vi "Overlay Geometric Pattern Matching Results.vi"(6 "Color":u32(colorbox)=16711680, 7 "Group":string, 8 "error in":errorcluster, 10 "Matches":T2[](array[typedef]) {"Correlation Score" format="%.2f"; "Target Template Curve Score" format="%.2f"; "Template Target Curve Score" format="%.2f"; "Bounding Box"."y" format="%.2f"; "Bounding Box"."x" format="%.2f"; "Position"."y" format="%.2f"; "Position"."x" format="%.2f"; "Score" format="%.2f"; "Scale" format="%.2f"; "Angle" format="%.2f"; "Occlusion %" format="%.2f"}, 11 "Image":T1) -> (0 "error out":errorcluster, 3 "Image Out":T1)   [LabVIEW 2014]
uses:
  <vilib>/vision/Pattern Matching.llb/IMAQ GM Match Report.ctl
  <vilib>/vision/Image Controls.llb/IMAQ Image.ctl
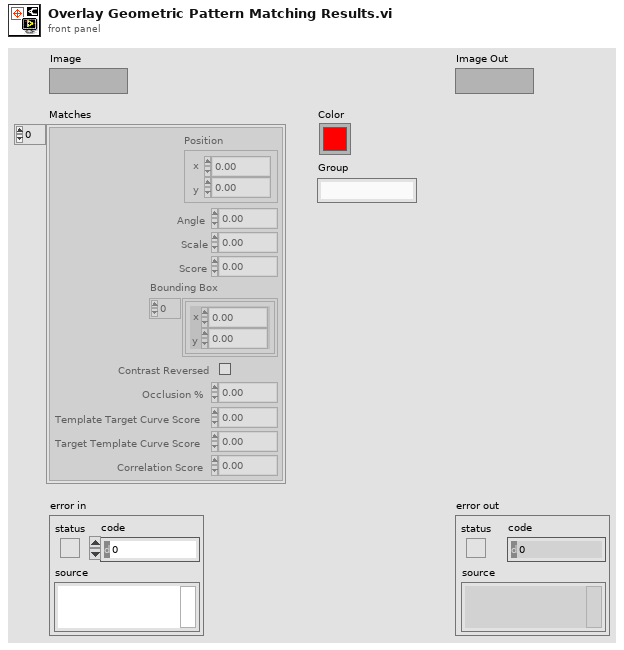
[diagram p1: front panel]
types:
  T1 = typedef "IMAQ Image.ctl" = refnum<image>
  T2 = typedef "IMAQ GM Match Report.ctl" = cluster{"Position":cluster{"x":sgl, "y":sgl}, "Angle":sgl, "Scale":sgl, "Score":sgl, "Bounding Box":cluster{"x":sgl, "y":sgl}[], "Contrast Reversed":bool, "Occlusion %":sgl, "Template Target Curve Score":sgl, "Target Template Curve Score":sgl, "Correlation Score":sgl}
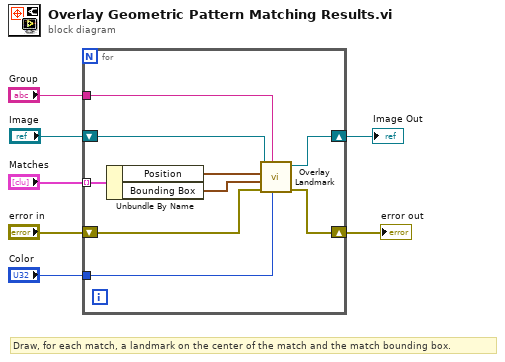
[diagram p0: block diagram]
diagram:
  # "Draw, for each match, a landmark on the center of the match and the match bounding box."
  n1 = for {
    shift-right: [w8] -> w1
    shift-left: "Image" -> [w15]
    tunnel: "Matches" -> [w16] mode=indexing
    tunnel: "Color" -> [w9]
    shift-right: [w10] -> w4
    shift-left: "error in" -> [w12]
    tunnel: "Group" -> [w14]
    n2 = Unbundle By Name(w16) -> ("Position"=w13:cluster{"x":sgl, "y":sgl}, "Bounding Box"=w11:cluster{"x":sgl, "y":sgl}[])
    n3 = call "Overlay Landmark.vi"("Color"=w9, "Group"=w14, "error in"=w12, "Bounding Box"=w11, "Position"=w13, "Image"=w15) -> ("error out"=w10:errorcluster, "Image Out"=w8:T1)  [unwired: 4 in]
  }
  "Image Out" <- w1
  "error out" <- w4
